vi "RunInference_U64.vi"(4 "Introspection Output":T1, 6 "outputIndex":i32, 8 "error in (no error)":errorcluster, 9 "inputIndex":i32, 10 "inputBuffer":sgl[](array[numeric]), 11 "session id in":i32) -> (0 "error out":errorcluster, 1 "Dims":i64[](array[numeric]), 2 "outputBuffer":u64[](array[numeric]), 3 "session id out":i32)   [LabVIEW 2017, in "libonnx_wrapper.lvlib"]
doc: "/**\n * @brief Выполнить инференс (предсказание) модели\n * \n * Основная функция для получения предсказания от модели. Принимает входные данные,\n * передаёт их в нейросеть и записывает результат в выходной буфер.\n * \n * @param sessionId [IN] ID сессии\n * @param inputIndex [IN] Индекс входа (обычно 0 для моделей с одним входом)\n * @param inputBuffer [IN] Массив входных данных (тип должен соответствовать GetInputType)\n * @param inputSize [IN] Количество элементов во входном массиве\n * @param outputIndex [IN] Индекс выхода (обычно 0 для моделей с одним выходом)\n * @param outputBuffer [OUT] Массив для записи результатов (должен быть выделен в LabVIEW)\n * @param outputSize [IN] Размер выходного буфера в элементах\n * \n * @return int32: 0 при успешном выполнении инференса\n * @return int32: -1 при ошибке (сессия не загружена, неверные индексы, ошибка ONNX Runtime)\n * \n * @note Входные данные должны быть нормализованы так же, как при обучении модели\n * @note Размер входного массива должен соответствовать произведению всех размерностей shape\n * @note Выходной буфер должен быть достаточного размера (см. GetOutputShapeDim)\n * @note Функция блокирует выполнение до завершения инференса\n * \n * @example\n * // Для модели с входом [1, 10] и выходом [1, 3]:\n * float inputData[10] = {...};\n * float outputData[3];\n * RunInference(sessionId, 0, inputData, 10, 0, outputData, 3);\n */\nint RunInference(int sessionId, int inputIndex, float* inputBuffer, int inputSize, \n int outputIndex, float* outputBuffer, int outputSize);"
uses:
  libonnx_wrapper.lvlib
  TypeDef/IO.ctl
  TypeDef/Introspection.ctl
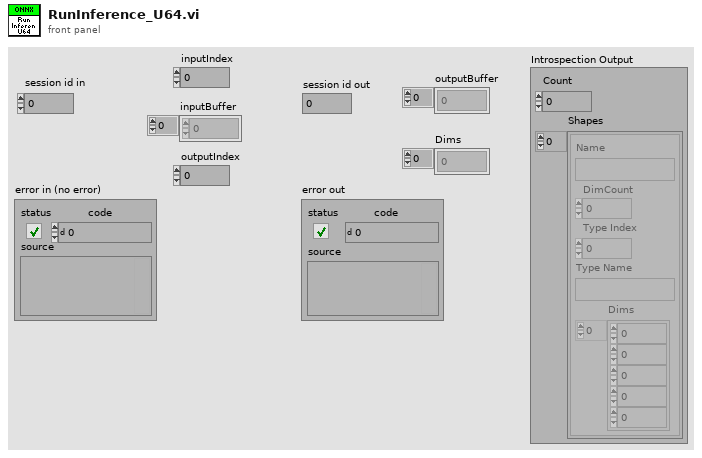
[diagram p1: front panel]
types:
  T1 = typedef "libonnx_wrapper.lvlib/Introspection.ctl" = cluster{"Count":i32, "Shapes":T2[]}
  T2 = typedef "libonnx_wrapper.lvlib/IO.ctl" = cluster{"Name":string, "DimCount":i32, "Type Index":i32, "Type Name":string, "Dims":i64[]}
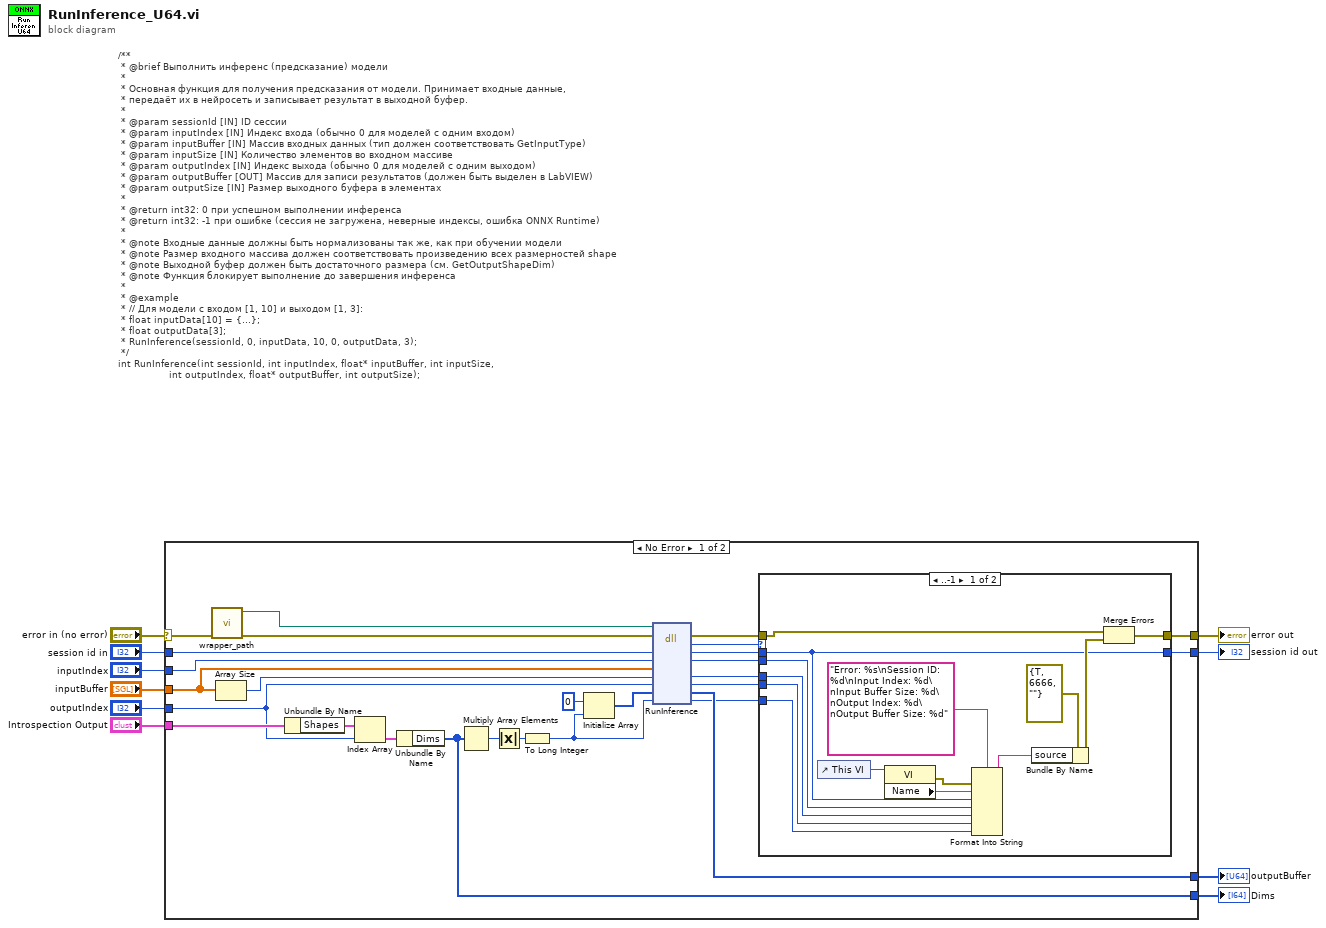
[diagram p0: block diagram]
diagram:
  # "/**\n * @brief Выполнить инференс (предсказание) модели\n * \n * Основная функция для получения предсказания от модели. Принимает входные данные,\n * передаёт их в нейросеть и записывает результат в выходной буфер.\n * \n * @param sessionId [IN] ID сессии\n * @param inputIndex [IN] Индекс входа (обычно 0 для моделей с одним входом)\n * @param inputBuffer [IN] Массив входных данных (тип должен соответствовать GetInputType)\n * @param inputSize [IN] Количество элементов во входном массиве\n * @param outputIndex [IN] Индекс выхода (обычно 0 для моделей с одним выходом)\n * @param outputBuffer [OUT] Массив для записи результатов (должен быть выделен в LabVIEW)\n * @param outputSize [IN] Размер выходного буфера в элементах\n * \n * @return int32: 0 при успешном выполнении инференса\n * @return int32: -1 при ошибке (сессия не загружена, неверные индексы, ошибка ONNX Runtime)\n * \n * @note Входные данные должны быть нормализованы так же, как при обучении модели\n * @note Размер входного массива должен соответствовать произведению всех размерностей shape\n * @note Выходной буфер должен быть достаточного размера (см. GetOutputShapeDim)\n * @note Функция блокирует выполнение до завершения инференса\n * \n * @example\n * // Для модели с входом [1, 10] и выходом [1, 3]:\n * float inputData[10] = {...};\n * float outputData[3];\n * RunInference(sessionId, 0, inputData, 10, 0, outputData, 3);\n */\nint RunInference(int sessionId, int inputIndex, float* inputBuffer, int inputSize, \n                 int outputIndex, float* outputBuffer, int outputSize);"
  n1 = case shown="No Error" "error in (no error)" {
    selector: "error in (no error)" -> [w11 w55]
    tunnel: "session id in" -> [w35 w54]
    tunnel: "inputIndex" -> [w34 _]
    tunnel: "inputBuffer" -> [w33 _]
    tunnel: [w29 _] -> w7
    tunnel: [w26 _] -> w6
    tunnel: "Introspection Output" -> [w22 _]
    tunnel: "outputIndex" -> [w21 _]
    tunnel: [w17 w55] -> w3
    tunnel: [w16 w54] -> w2
    frame No Error {
      n2 = call "wrapper_path.vi"("error in (no error)"=w11) -> ("error out"=w36:errorcluster, "wrapper path"=w37:path)  [unwired: 9 in]
      n3 = Array Size(array=w33) -> (size(s)=w32:i32)
      n4 = Unbundle By Name(w22) -> ("Shapes"=w28:T2[])
      n5 = Index Array(array=w28, index=w21) -> (element=w27:T2)
      n6 = Unbundle By Name(w27) -> ("Dims"=w26:i64[])
      n7 = Multiply Array Elements(1:w26) -> (0:w25:i64)
      n8 = Absolute Value(x=w25) -> (abs(x)=w24:i64)
      n9 = To Long Integer(number=w24) -> (32bit integer=w23:i32)
      n10 = Initialize Array(u64 0 ("element"), w23) -> (w30:u64[])
      n11 = dll-call lib="home/ivan/LabVIEWData/ONNX/Test/libonnx_wrapper/unix64/libonnx_wrapper.*" fn="RunInference"(path in=w37, error in=w36, "sessionId"=w35, "inputIndex"=w34, "inputBuffer"=w33, "inputSize"=w32, "outputIndex"=w21, "outputBuffer"=w30, "outputSize"=w23) -> (error out=w20:errorcluster, "return"=w19:i32, "sessionId"=w18:i32, "inputIndex"=w15:i32, "inputSize"=w14:i32, "outputIndex"=w13:i32, "outputBuffer"=w29:u64[], "outputSize"=w12:i32)  [unwired: 2 in, 1 out]
      n12 = case shown="..-1" w19 {
        tunnel: w20 -> [w42 w53]
        tunnel: [w43 w53] -> w17
        tunnel: w18 -> [w44 w52]
        tunnel: [w44 w52] -> w16
        tunnel: w15 -> [w41 _]
        tunnel: w14 -> [w40 _]
        tunnel: w13 -> [w39 _]
        tunnel: w12 -> [w38 _]
        frame ..-1 {
          n13 = control-ref of="This VI"() -> (w48:refnum<vi>)
          n14 = property class="VI"(reference=w48) -> (error out=w45:errorcluster, "Name"=w47:string)  [unwired: 1 in, 1 out]
          n15 = Format Into String(format string="Error: %s\nSession ID: %d\nInput Index: %d\nInput Buffer Size: %d\nOutput Index: %d\nOutput Buffer Size: %d", error in=w45, w47, w44, w41, w40, w39, w38) -> (resulting string=w49:string)  [unwired: 1 in, 1 out]
          n16 = Bundle By Name(cluster=errorcluster {"status"=TRUE, "code"=6666, "source"=""} ("error out"), "source"=w49) -> (w50:errorcluster)
          n17 = Merge Errors(w42, w50) -> (w43:errorcluster)
        }
        frame 0.. {
        }
      }
    }
    frame Error {
    }
  }
  "error out" <- w3
  "session id out" <- w2
  "outputBuffer" <- w7
  "Dims" <- w6
